vi "conversion.vi"(8 "map":u16[][](array[numeric]), 10 "c":i32, 11 "r":i32) -> (2 "c":i32, 3 "r":i32)   [LabVIEW 2014]
doc: "convert the nonexisting coordination to proper coordination"
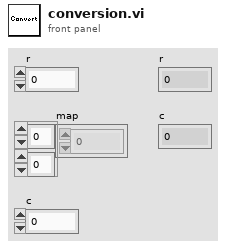
[diagram p1: front panel]
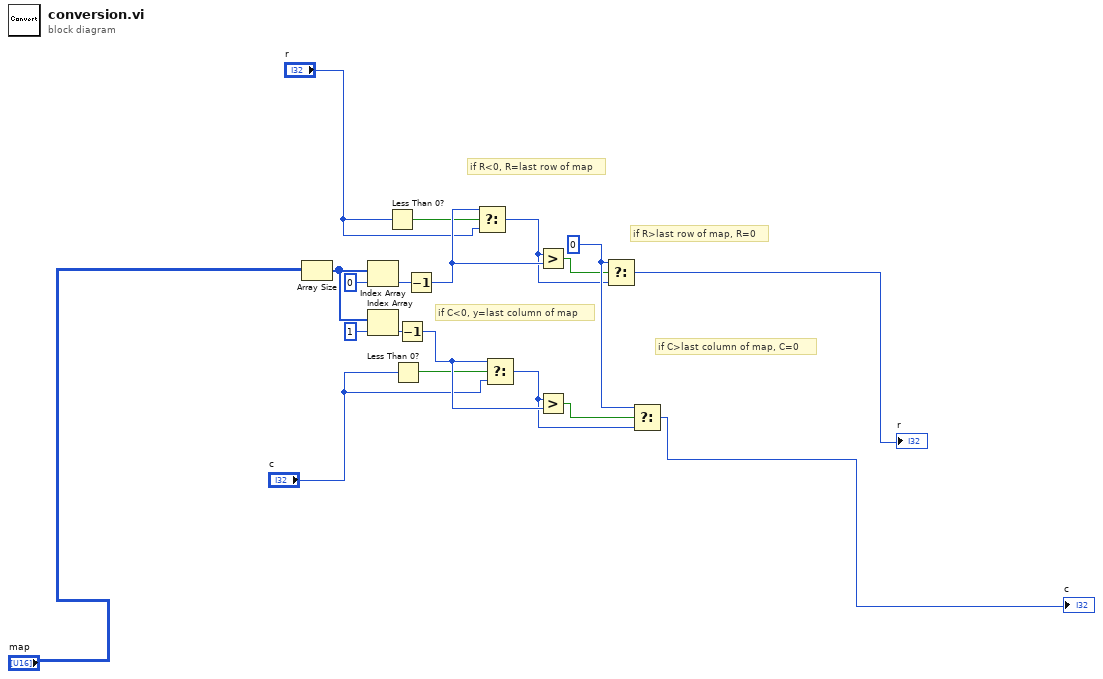
[diagram p0: block diagram]
diagram:
  w14 = 0 ("index")
  # "if C>last column of map, C=0"
  # "if C<0, y=last column of map"
  # "if R>last row of map, R=0"
  # "if R<0, R=last row of map"
  n1 = Array Size(array="map") -> (size(s)=w3:i32[])
  n2 = Index Array(array=w3, index=0) -> (element=w6:i32)
  n3 = Index Array(array=w3, index=1) -> (element=w12:i32)
  n4 = Less Than 0?(x="r") -> (x < 0?=w1:bool)
  n5 = Less Than 0?(x="c") -> (x < 0?=w10:bool)
  n6 = Decrement(x=w12) -> (x-1=w18:i32)
  n7 = Decrement(x=w6) -> (x-1=w17:i32)
  n8 = Select(t=w17, s=w1, f="r") -> (s? t:f=w8:i32)
  n9 = Select(t=w18, s=w10, f="c") -> (s? t:f=w15:i32)
  n10 = Greater?(x=w8, y=w17) -> (0:w7:bool)
  n11 = Greater?(x=w15, y=w18) -> (0:w13:bool)
  n12 = Select(t=w14, s=w7, f=w8) -> (s? t:f=→"r":i32)
  n13 = Select(t=w14, s=w13, f=w15) -> (s? t:f=→"c":i32)
